vi "Turn Generator Off.vi"(8 "error in (no error)":errorcluster, 11 "Arinst SSA-TG in":refnum<class "PL Arinst SSA-TG.lvclass">) -> (0 "error out":errorcluster, 3 "Arinst SSA-TG out":refnum<class "PL Arinst SSA-TG.lvclass">)   [LabVIEW 2015, in "PL Arinst SSA-TG.lvclass"]
doc: "Turns generator off."
uses:
  PL Arinst SSA-TG.lvclass
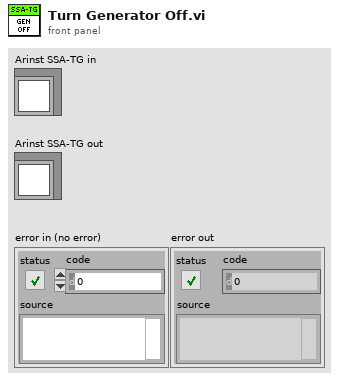
[diagram p1: front panel]
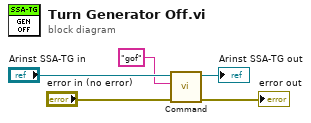
[diagram p0: block diagram]
diagram:
  n1 = call "Command.vi"("error in (no error)"="error in (no error)", "command"="gof", "Arinst SSA-TG in"="Arinst SSA-TG in") -> ("error out"=→"error out":errorcluster, "Arinst SSA-TG out"=→"Arinst SSA-TG out":refnum<class "PL Arinst SSA-TG.lvclass">)  [unwired: 6 in, 1 out]
